vi "Sound-PlayTone.vi"(4 "df Array":dbl[](array[numeric]), 5 "sound?":bool, 6 "# samples":u32, 7 "Sound Controls":T2={"device ID"=0, "sound format"={"sample rate (S/s)"=44000.0, "number of channels"=2, "bits per sample"=16}, "time (ms)"=200.0}, 8 "Frecuencia":dbl, 9 "Sound Device IN":T4 {"task ID" format="%.0x"}) -> (0 "Waveform":waveform(dbl), 3 "Sound Device OUT":T4 {"task ID" format="%.0x"})   [LabVIEW 2010]
uses:
  <vilib>/sound2/lvsound2.llb/Sound Output Task ID.ctl
  <vilib>/sound2/lvsound2.llb/Sound Data Format.ctl
  <vilib>/sound2/lvsound2.llb/Sound Output Write (DBL Single).vi
panel:
  out "Waveform Graph":waveform(dbl)(graph)
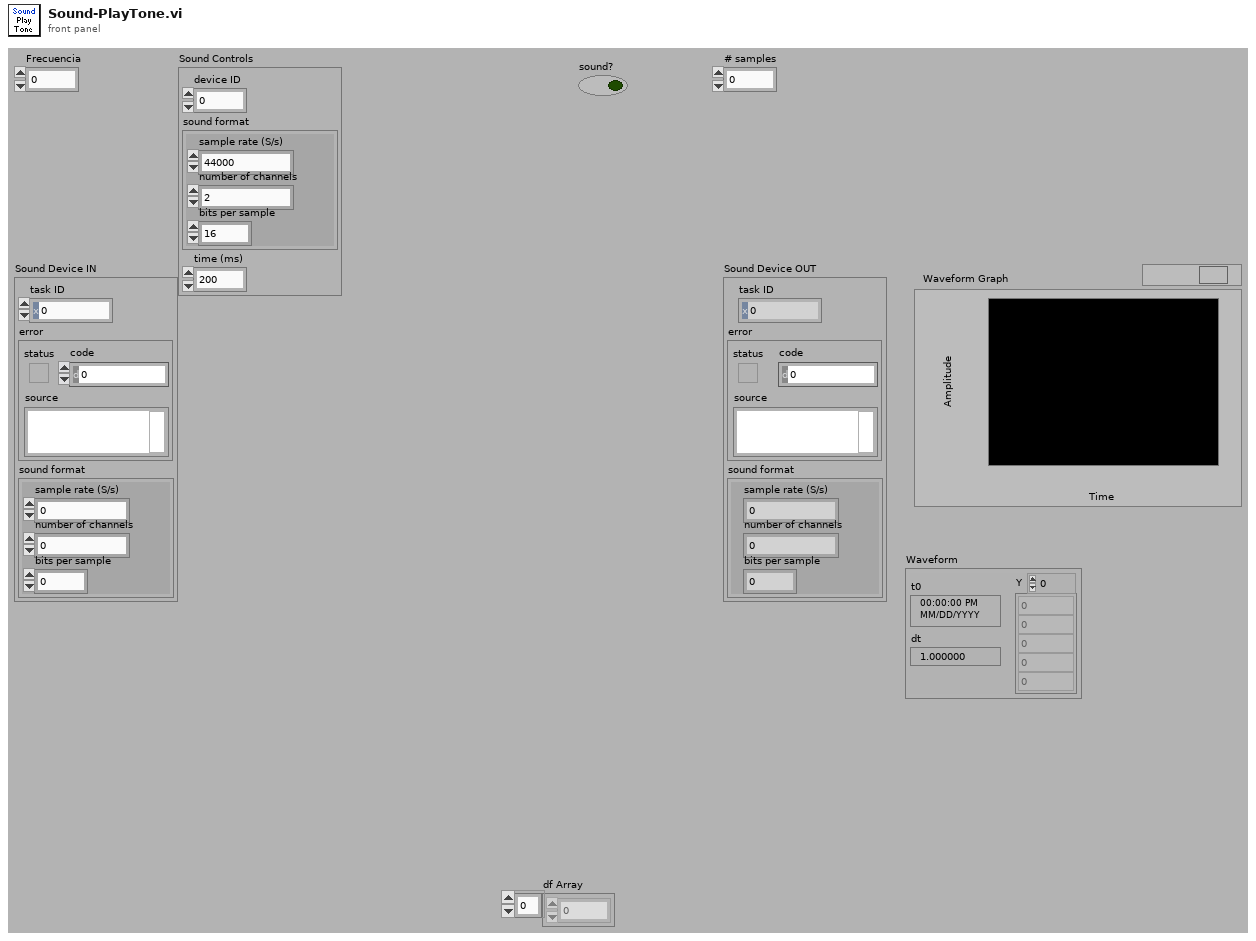
[diagram p1: front panel]
types:
  T1 = typedef "Sound Data Format.ctl" = cluster{"sample rate (S/s)":dbl, "number of channels":i32, "bits per sample":i32}
  T2 = cluster{"device ID":u32, "sound format":T1, "time (ms)":dbl}
  T3 = typedef "Sound Output Task ID.ctl" = u32
  T4 = cluster{"task ID":T3, "error":errorcluster, "sound format":T1}
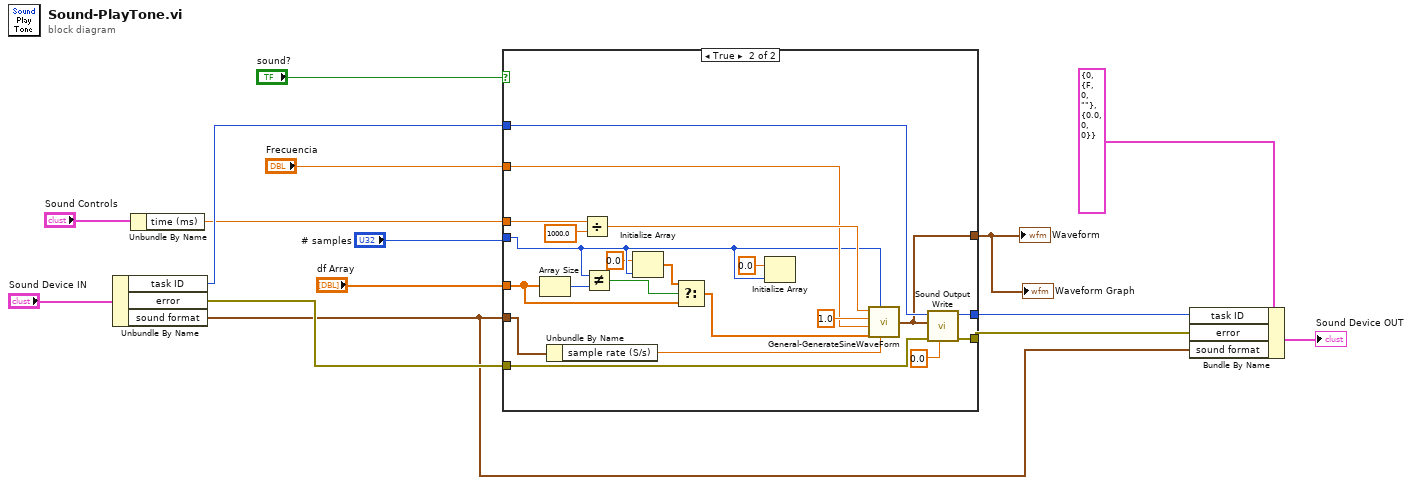
[diagram p0: block diagram]
diagram:
  n1 = Unbundle By Name("Sound Device IN") -> ("task ID"=w13:T3, "error"=w12:errorcluster, "sound format"=w6:T1)
  n2 = Unbundle By Name("Sound Controls") -> ("time (ms)"=w2:dbl)
  n3 = case shown="True" "sound?" {
    tunnel: w13 -> [w16 w38]
    tunnel: [w16 w37] -> w11
    tunnel: w12 -> [w17 w36]
    tunnel: [w17 w35] -> w10
    tunnel: w6 -> [_ w33]
    tunnel: w2 -> [_ w30]
    tunnel: "df Array" -> [_ w23]
    tunnel: "# samples" -> [_ w19]
    tunnel: [_ w27] -> w5
    tunnel: "Frecuencia" -> [_ w25]
    frame False {
    }
    frame True {
      n4 = Array Size(array=w23) -> (size(s)=w24:i32)
      n5 = Unbundle By Name(w33) -> ("sample rate (S/s)"=w29:dbl)
      n6 = Divide(x=w30, y=1000.0) -> (x/y=w28:dbl)
      n7 = Not Equal?(x=w19, y=w24) -> (x != y?=w22:bool)
      n8 = Initialize Array(0.0 ("element"), w19) -> (w20:dbl[])
      n9 = Select(t=w20, s=w22, f=w23) -> (s? t:f=w21:dbl[])
      n10 = Initialize Array(0.0 ("element"), w19) -> ()  [unwired: 1 out]
      n11 = call "General-GenerateSineWaveForm.vi"("tiempo (s)"=w28, "#samples"=w19, "Amplitud"=1.0, "frecuencia"=w25, "Fs (S/s)"=w29, "df"=w21) -> ("Waveform"=w27:waveform(dbl))  [unwired: 2 in]
      n12 = call-poly <vilib>:"Sound Output Write.vi"("timeout (sec)"=0.0, "error in (no error)"=w36, "data"=w27, "task ID"=w38) -> ("error out"=w35:errorcluster, "task ID out"=w37:T3)  [unwired: 6 in]
    }
  }
  "Waveform" <- w5
  "Waveform Graph" <- w5
  n13 = Bundle By Name(cluster=T4 {"task ID"=0, "error"={"status"=FALSE, "code"=0, "source"=""}, "sound format"={"sample rate (S/s)"=0.0, "number of channels"=0, "bits per sample"=0}} ("Sound Device IN"), "task ID"=w11, "error"=w10, "sound format"=w6) -> (→"Sound Device OUT":T4)
